vi "SetMotors_with_PID(SUBVI).vi"(10 "steering frame velocity":dbl[](array[numeric])=[0.0, 0.0, 0.0], 11 "Reset Encoders":bool) -> (1 "Vasen":cluster{"initial PV":dbl, "SP:":dbl}(graph)={"initial PV"=0.0, "SP:"=-0.0}, 2 "Taka":cluster{"initial PV":dbl, "SP:":dbl}(graph)={"initial PV"=0.0, "SP:"=-0.0}, 3 "Etu":cluster{"initial PV":dbl, "SP:":dbl}(graph)={"initial PV"=0.0, "SP:"=-0.0}, 4 "Oikea":cluster{"initial PV":dbl, "SP:":dbl}(graph)={"initial PV"=0.0, "SP:"=-0.0}, 5 "Radians/s":dbl[](array[numeric]), 6 "ccw motor velocity setpoints":dbl[](array[numeric])=[-0.0, -0.0, -0.0, -0.0])   [LabVIEW 2018]
uses:
  <vilib>/robotics/Steering/Wheel/Wheel Parameters.ctl
  <vilib>/robotics/Steering/Wheel/Rotation Direction.ctl
  <vilib>/robotics/Steering/Omnidirectional Wheel/NI_Robotics_Omnidirectional Wheel.lvclass
  C:/Program Files (x86)/National Instruments/LabVIEW 2018/vi.lib/robotics/Steering/Wheel/NI_Robotics_Wheel.lvclass
  <vilib>/robotics/Steering/Omnidirectional Wheel/Create Omnidirectional Wheel.vi
  <vilib>/robotics/Steering/Steering Frame/Create User Defined Steering Frame.vi
  <vilib>/robotics/Steering/Steering Frame/Apply Steering Frame Velocity to Motors.vi
  <vilib>/addons/control/pid/pid.llb/PID (DBL Array).vi
  <vilib>/robotics/Steering/Create Steering Frame/NI_Robotics_Create Steering Frame.xnode
  <vilib>/robotics/Steering/Class Type Definitions/Steering Frame.ctl
  <vilib>/robotics/Steering/Steering Frame/NI_Robotics_Steering Frame.lvclass
  <vilib>/addons/control/pid/NI_PID_pid.lvlib
  <vilib>/robotics/Steering/Class Type Definitions/NI_Robotics_Steering Class Types.lvlib
  <vilib>/robotics/Steering/Wheel/NI_Robotics_Wheel.lvclass
panel:
  in  "PID gains":T1(array[cluster])=[{"proportional gain (Kc)"=1.0, "integral time (Ti, min)"=0.01, "derivative time (Td, min)"=0.0}] {"derivative time (Td, min)" format="%.3f"; "integral time (Ti, min)" format="%.3f"; "proportional gain (Kc)" format="%.3f"}
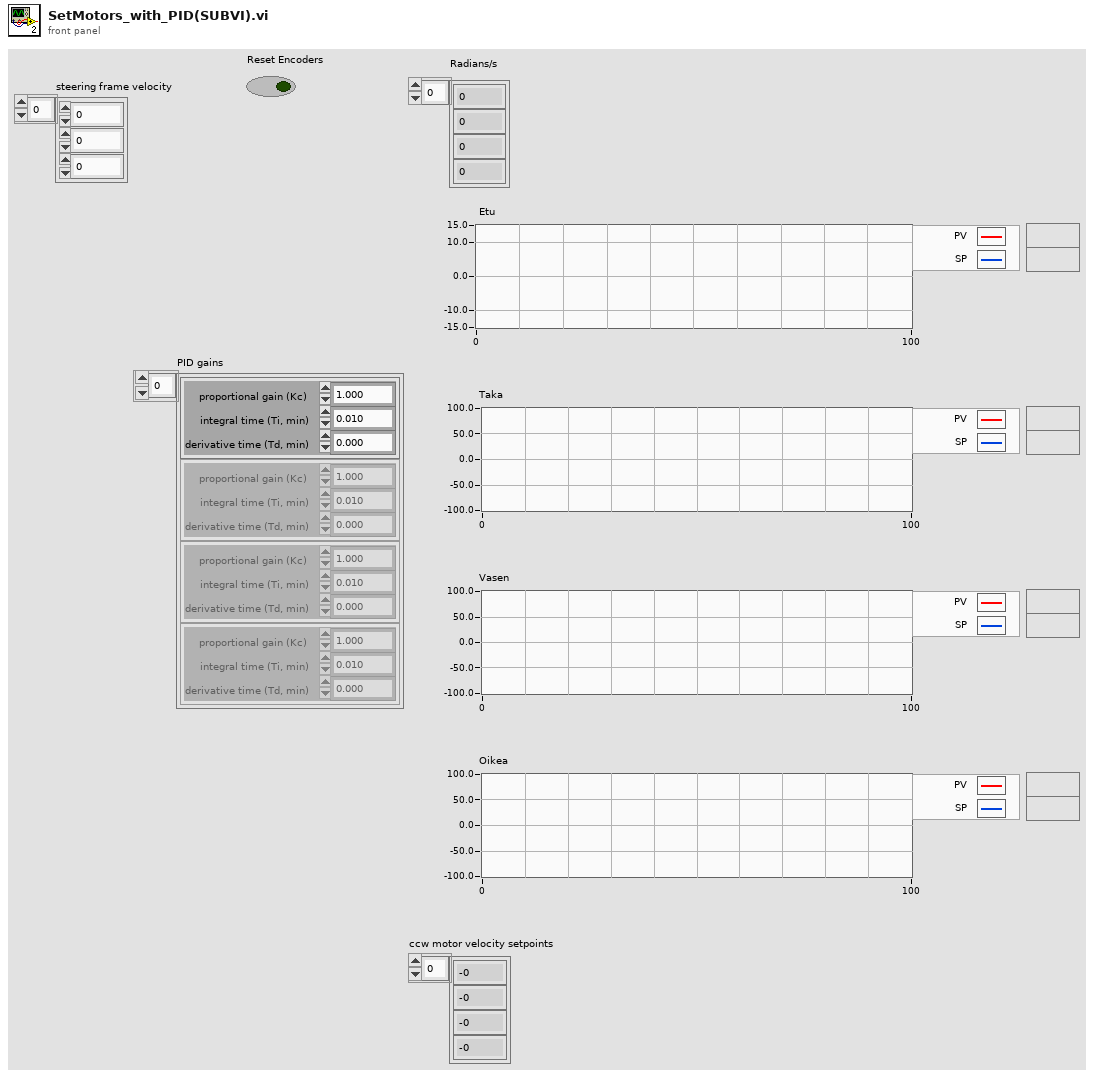
[diagram p1: front panel]
types:
  T1 = cluster{"proportional gain (Kc)":dbl, "integral time (Ti, min)":dbl, "derivative time (Td, min)":dbl}[]
  T2 = cluster{bool, "Tick Count(uSec)":u32, "Counter Value":i32[], "x-y":i32[]}
  T3 = typedef "NI_Robotics_Steering Class Types.lvlib/Steering Frame.ctl" = refnum<class "NI_Robotics_Steering Frame.lvclass">
  T4 = cluster{"Position":i32[], "Velocity RPM":dbl[], "Velocity RPS":dbl[], "Radians/s":dbl[]}
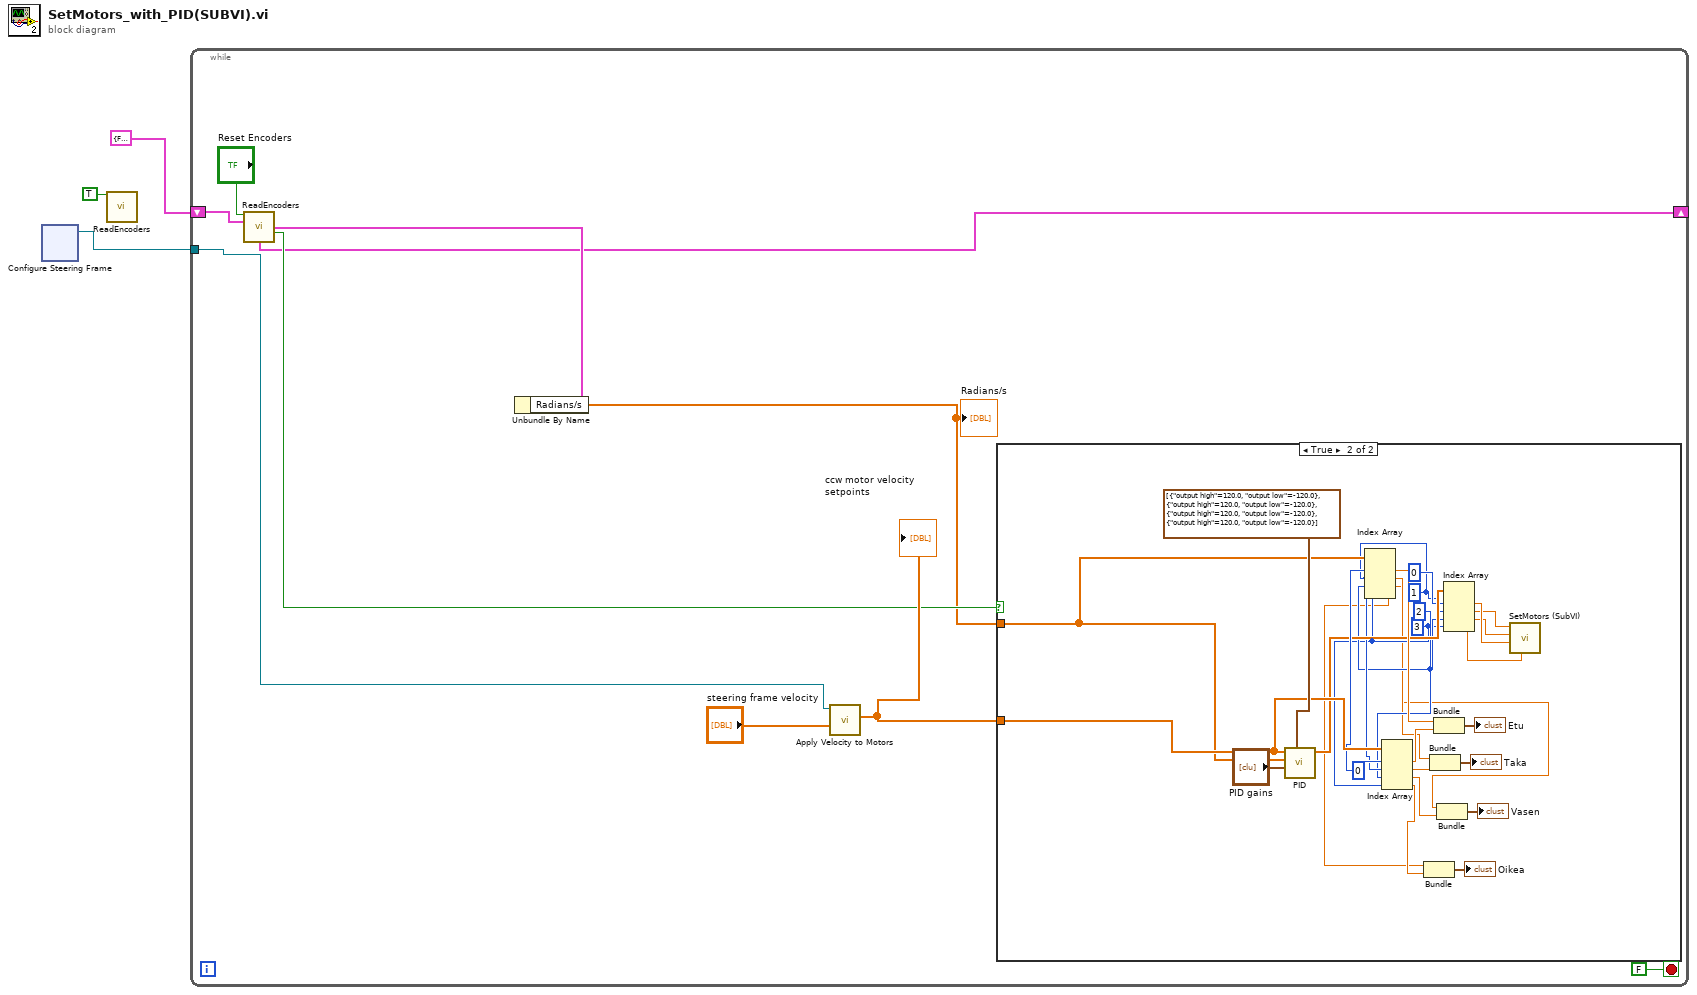
[diagram p0: block diagram]
diagram:
  n1 = xnode ("Configure Steering Frame")() -> ("steering frame out"=w2:T3)  [unwired: 1 in, 1 out]
  n2 = call "ReadEncoders.vi"("Reset Encoders"=TRUE) -> ()  [unwired: 10 in, 5 out]
  n3 = while {
    tunnel: w2 -> [w12]
    shift-right: [w5] -> _
    shift-left: T2 {FALSE, "Tick Count(uSec)"=0, "Counter Value"=[0, 0, 0, 0], "x-y"=[0, 0, 0, 0]} ("Cluster in") -> [w13]
    stop <- FALSE stop-if-true
    n4 = call "ReadEncoders.vi"("Reset Encoders"="Reset Encoders", "Cluster in"=w13) -> ("output cluster"=w9:T4, "Cluster Out"=w5:T2, "Updated"=w8:bool)  [unwired: 9 in, 2 out]
    n5 = Unbundle By Name(w9) -> ("Radians/s"=w7:dbl[])
    "Radians/s" <- w7
    n6 = call-poly <vilib>:"Apply Velocity to Motors.vi"("steering frame velocity"="steering frame velocity", "steering frame in"=w12) -> ("ccw motor velocity setpoints"=w10:dbl[])  [unwired: 5 in, 4 out]
    "ccw motor velocity setpoints" <- w10
    n7 = case shown="True" w8 {
      tunnel: w10 -> [_ w38]
      tunnel: w7 -> [_ w33]
      frame False {
      }
      frame True {
        w18 = 3 ("index")
        w19 = 2 ("index")
        w20 = 1 ("index")
        w37 = 0 ("index")
        n8 = call-poly <vilib>:"PID.vi"("output range"=cluster{"output high":dbl, "output low":dbl}[] [{"output high"=120.0, "output low"=-120.0}, {"output high"=120.0, "output low"=-120.0}, {"output high"=120.0, "output low"=-120.0}, {"output high"=120.0, "output low"=-120.0}], "PID gains"="PID gains", "process variable"=w33, "setpoint"=w38) -> ("output"=w32:dbl[])  [unwired: 6 in, 1 out]
        n9 = Index Array(array=w33, index #1=w37, index #2=w20, index #3=w19, index #4=w18) -> (element #1=w35:dbl, element #2=w17:dbl, element #3=w16:dbl, element #4=w15:dbl)
        n10 = Index Array(array=w38, index #1=w37, index #2=w20, index #3=w19, index #4=w18) -> (element #1=w34:dbl, element #2=w21:dbl, element #3=w22:dbl, element #4=w23:dbl)
        n11 = Bundle(w15, "Numeric"=w23) -> (→"Oikea":cluster{dbl, "Numeric":dbl})  [unwired: 1 in]
        n12 = Bundle(w17, "Numeric"=w21) -> (→"Taka":cluster{dbl, "Numeric":dbl})  [unwired: 1 in]
        n13 = Bundle(w35, "Numeric"=w34) -> (→"Etu":cluster{dbl, "Numeric":dbl})  [unwired: 1 in]
        n14 = Bundle(w16, "Numeric"=w22) -> (→"Vasen":cluster{dbl, "Numeric":dbl})  [unwired: 1 in]
        n15 = Index Array(array=w32, index #1=0 ("index"), index #2=w20, index #3=w19, index #4=w18) -> (element #1=w30:dbl, element #2=w29:dbl, element #3=w28:dbl, element #4=w27:dbl)
        n16 = call "SetMotors (SubVI).vi"("Oikea"=w27, "Etu"=w30, "Vasen"=w28, "Taka"=w29) -> ()  [unwired: 8 in]
      }
    }
  }
